vi "Unflatten Compiled Data.vi"(8 "error in (no error)":errorcluster, 9 "Compiled.Settings":T5 {"Execution Unit Compiled Information"."Outgoing Data References"."Data Reference" format="%.0x"; "Execution Unit Compiled Information"."Incoming Data References" format="%.0x"}, 10 "RT State Variables in":T1 {"Execution Unit Runtime Information"."Outgoing Data References"."Data Reference" format="%.0x"; "Execution Unit Runtime Information"."Incoming Data References" format="%.0x"}, 11 "Item Ref in":T7 format="%.0x") -> (0 "error out":errorcluster, 2 "RT State Variables out":T1 {"Execution Unit Runtime Information"."Outgoing Data References"."Data Reference" format="%.0x"; "Execution Unit Runtime Information"."Incoming Data References" format="%.0x"}, 3 "Item Ref out":T7 format="%.0x")   [LabVIEW 2020, in "Communication Bus Template Engine.lvlib"]
uses:
  Communication Bus Template Engine.lvlib
  Includes/Communication Bus Interfaces.lvlibp/Execution Unit/Execution Unit/Execution Unit.lvclass
  <vilib>/NI VeriStand/Custom Device API/Custom Device Item Ref.ctl
  <vilib>/NI VeriStand/Custom Device API/Custom Device API.lvlib
  <vilib>/NI VeriStand/Custom Device API/Data Reference.ctl
  <vilib>/NI VeriStand/Custom Device API/Block Data Reference.ctl
  Shared/Execution Unit Compiled Information.ctl
  Shared/Communication Bus Template Shared.lvlib
  Shared/Compiled.Settings.ctl
  <vilib>/NI/NIVS Inline Async API/_VS Inline Async API/VS Inline Async API/VS Inline Async API.lvclass
  RTStateVariables.ctl
  Execution Unit Runtime Information.ctl
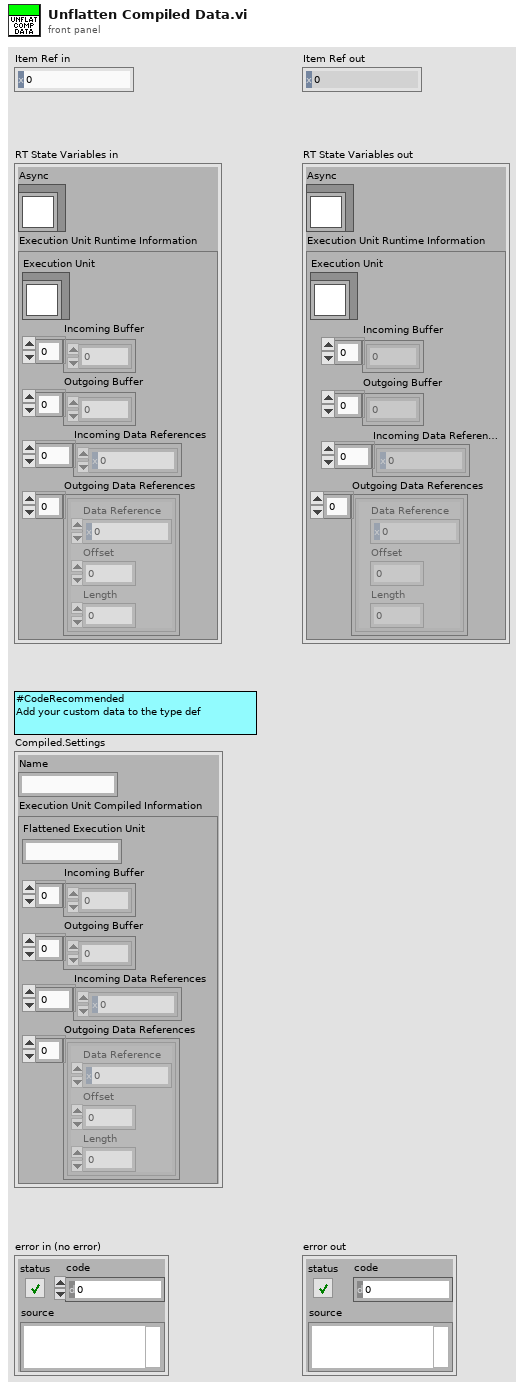
[diagram p1: front panel]
types:
  T1 = typedef "Communication Bus Template Engine.lvlib/RTStateVariables.ctl" = cluster{"Async":refnum<class "VS Inline Async API.lvclass">, "Execution Unit Runtime Information":T2}
  T2 = typedef "Communication Bus Template Engine.lvlib/Execution Unit Runtime Information.ctl" = cluster{"Execution Unit":refnum<class "Execution Unit.lvclass">, "Incoming Buffer":dbl[], "Outgoing Buffer":dbl[], "Incoming Data References":T3[], "Outgoing Data References":T4[]}
  T3 = typedef "Custom Device API.lvlib/Data Reference.ctl" = i32
  T4 = typedef "Custom Device API.lvlib/Block Data Reference.ctl" = cluster{"Data Reference":T3, "Offset":u64, "Length":u64}
  T5 = typedef "Communication Bus Template Shared.lvlib/Compiled.Settings.ctl" = cluster{"Name":string, "Execution Unit Compiled Information":T6}
  T6 = typedef "Communication Bus Template Shared.lvlib/Execution Unit Compiled Information.ctl" = cluster{"Flattened Execution Unit":string, "Incoming Buffer":dbl[], "Outgoing Buffer":dbl[], "Incoming Data References":T3[], "Outgoing Data References":T4[]}
  T7 = typedef "Custom Device API.lvlib/Custom Device Item Ref.ctl" = u64
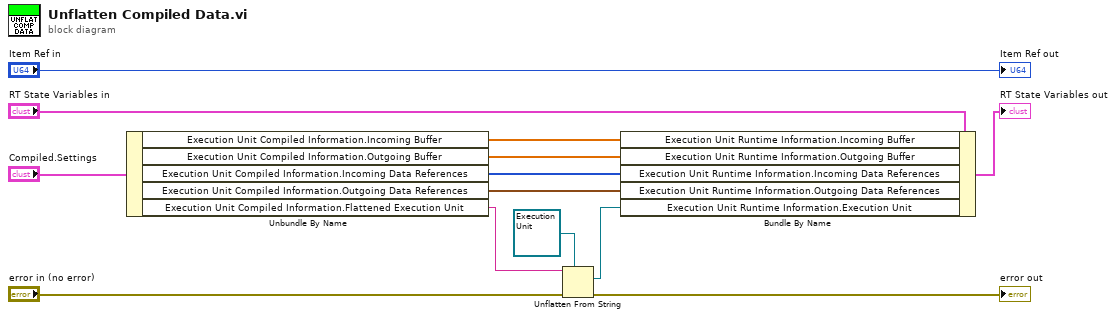
[diagram p0: block diagram]
diagram:
  n1 = Unbundle By Name("Compiled.Settings") -> ("Execution Unit Compiled Information.Incoming Buffer"=w7:dbl[], "Execution Unit Compiled Information.Outgoing Buffer"=w6:dbl[], "Execution Unit Compiled Information.Incoming Data References"=w5:T3[], "Execution Unit Compiled Information.Outgoing Data References"=w4:T4[], "Execution Unit Compiled Information.Flattened Execution Unit"=w2:string)
  n2 = Unflatten From String(type=refnum<class "Execution Unit.lvclass"> refnum ("Communication Bus Template Interfaces:Execution Unit.lvlib:Execution Unit.lvclass"), binary string=w2, error in (no error)="error in (no error)") -> (value=w1:refnum<class "Execution Unit.lvclass">, error out=→"error out":errorcluster)  [unwired: 2 in, 1 out]
  n3 = Bundle By Name(cluster="RT State Variables in", "Execution Unit Runtime Information.Incoming Buffer"=w7, "Execution Unit Runtime Information.Outgoing Buffer"=w6, "Execution Unit Runtime Information.Incoming Data References"=w5, "Execution Unit Runtime Information.Outgoing Data References"=w4, "Execution Unit Runtime Information.Execution Unit"=w1) -> (→"RT State Variables out":T1)
  "Item Ref out" <- "Item Ref in"
